vi "sub VI example.vi"() -> ()   [LabVIEW 2024]
panel:
  in  "Slide":i64(slide) scale=0.0..120.0
  out "Thermometer":dbl(slide) scale=0.0..100.0
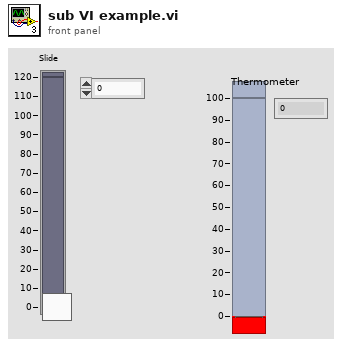
[diagram p1: front panel]
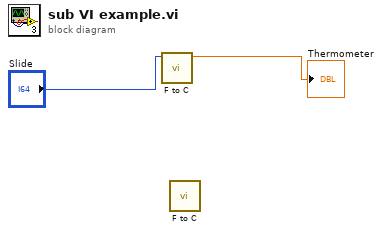
[diagram p0: block diagram]
diagram:
  n1 = call "F to C.vi"("Slide"="Slide") -> ("Numeric"=→"Thermometer":dbl)  [unwired: 10 in]
  n2 = call "F to C.vi"() -> ()  [unwired: 11 in, 1 out]
